vi "Handle Last Ack Core.vi"(4 "error in (no error)":errorcluster, 6 "Last Ack":refnum<class "Last Ack.lvclass">, 7 "Parallelizer in":refnum<class "Parallelizer.lvclass">) -> (0 "error out":errorcluster, 3 "Parallelizer out":refnum<class "Parallelizer.lvclass">)   [LabVIEW 2017, in "Parallelizer Example.lvlib" / "Parallelizer.lvclass"]
doc: "(<B>Filename</B>: Actor Framework.lvlib:Actor.lvclass:Handle Last Ack Core.vi)\n\nDefines how the caller actor responds to the Last Ack message from a nested actor. The Last Ack message is the final message a nested actor sends to its caller before it shuts down. The message contains information about the final state of the nested actor.\n\nBy default, this method does nothing except return any error the nested actor sent. A descendant class may override this method to define behavior."
uses:
  <vilib>/gpm_packages/@cs/test-executive/Source/Sandbox/Parallelizer Example/Parallelizer/Parallelizer.lvclass
  <vilib>/ActorFramework/LastAck/Last Ack.lvclass
  C:/Program Files/National Instruments/LabVIEW 2017/vi.lib/ActorFramework/Actor/Actor.lvclass
  <vilib>/gpm_packages/@cs/test-executive/Source/Sandbox/Parallelizer Example/Parallelizer/Parallelizer.lvclass/Parallelizer.ctl
  <vilib>/ActorFramework/Actor/Actor.lvclass/Actor.ctl
  <vilib>/ActorFramework/Message Enqueuer/Message Enqueuer.lvclass/Message Enqueuer.ctl
  <vilib>/ActorFramework/Message Enqueuer/Init from Existing Queue.vi
  <vilib>/ActorFramework/Message Enqueuer/Enqueue.vi
  <vilib>/ActorFramework/Stop Msg/Stop Msg.lvclass
  C:/Program Files/National Instruments/LabVIEW 2017/vi.lib/ActorFramework/Message/Message.lvclass
  <vilib>/ActorFramework/Message Priority Queue/Priority Enqueue.vi
  <vilib>/gpm_packages/@cs/test-executive/Source/Sandbox/Parallelizer Example/iTest Step/iTest Step.lvclass
  <vilib>/ActorFramework/Message Enqueuer/Message Enqueuer.lvclass
  <vilib>/ActorFramework/Actor/Actor.lvclass
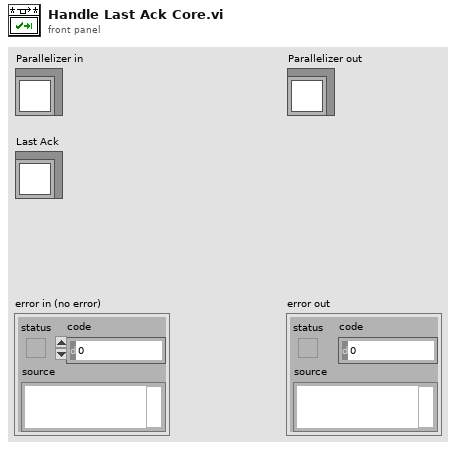
[diagram p1: front panel]
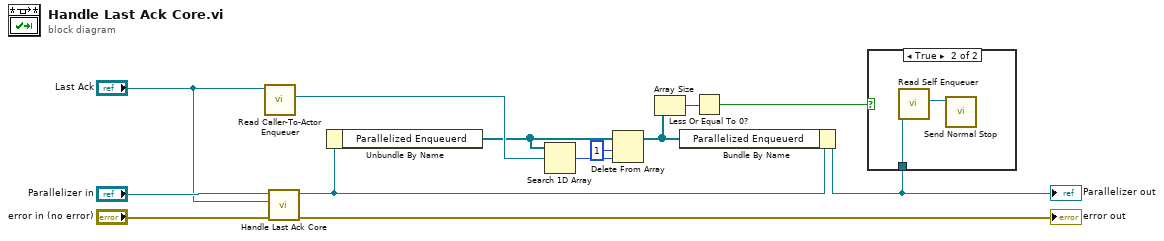
[diagram p0: block diagram]
diagram:
  n1 = call <vilib>:"Read Caller-To-Actor Enqueuer.vi"("Last Ack"="Last Ack") -> ("Caller-to-Actor Enqueuer"=w9:refnum<class "Message Enqueuer.lvclass">)  [unwired: 10 in]
  n2 = call-parent "Handle Last Ack Core.vi"("error in (no error)"="error in (no error)", "Last Ack"="Last Ack", "Actor in"="Parallelizer in") -> ("error out"=→"error out":errorcluster, "Actor out"=w5:refnum<class "Parallelizer.lvclass">)  [unwired: 3 in]
  n3 = Unbundle By Name(w5) -> ("Parallelized Enqueuerd"=w8:refnum<class "Message Enqueuer.lvclass">[])
  n4 = Search 1D Array(1D array=w8, element=w9) -> (index of element=w7:i32)  [unwired: 1 in]
  n5 = Delete From Array(array=w8, length=1, index=w7) -> (array with subset deleted=w4:refnum<class "Message Enqueuer.lvclass">[])  [unwired: 1 out]
  n6 = Array Size(array=w4) -> (size(s)=w3:i32)
  n7 = Bundle By Name(cluster=w5, "Parallelized Enqueuerd"=w4) -> (w2:refnum<class "Parallelizer.lvclass">)
  "Parallelizer out" <- w2
  n8 = Less Or Equal To 0?(x=w3) -> (x <= 0?=w1:bool)
  n9 = case shown="True" w1 {
    tunnel: w2 -> [_ w15]
    frame False {
    }
    frame True {
      n10 = call <vilib>:"Read Self Enqueuer.vi"("Actor"=w15) -> ("Self Enqueuer"=w14:refnum<class "Message Enqueuer.lvclass">)  [unwired: 10 in]
      n11 = call <vilib>:"Send Normal Stop.vi"("Message Enqueuer"=w14) -> ()  [unwired: 10 in, 1 out]
    }
  }
